vi "InitializeAllConfigs.vi"(10 "AllControlsRefs":T1, 11 "InstruConfig":T2={"Mode"="", "InstrumentMode"={"MainDAQ_Selector"=enum."None", "LaserCtrlMethod"=enum."SRS_DG535", "InstruMode"=enum."fsLDPI"}, "CommuniationSettings"={"SDG_II"="", "DG535"="", "BNC565"="", "EPM2000"="", "NI-DAQmx"="", "Micos"={"Simulation"=FALSE, "ComPort"="", "Serial Config"={"Baud Rate"=0, "Parity"=0, "Data Bits"=0, "Stop Bits"=0, "Flow Control"=0}, "#Axis"=0}, "ESP300"={"Simulation"=FALSE, "ComPort"="", "Serial Config"={"Baud Rate"=0, "Parity"=0, "Data Bits"=0, "Stop Bits"=0, "Flow Control"=0}, "#Axis"=0}}, "DG535"={"Trigger"={"Trigger Mode"=enum."Internal", "Internal/Burst Rate"=0.0, "External  Level"=0.0, "Impedance"=FALSE, "Slope"=FALSE}, "Delays"=[], "Output"=[]}, "Gage_Config"={"Acquisition"={"Sample Rate"=0.0, "Mode"=0, "Start (0)"=0.0, "Depth"=0.0, "Segment Size"=0.0, "Trigger Delay"=0.0, "Trigger Timeout"=0.0, "Trigger Holdoff"=0.0, "Clock mode"=enum."Internal", "Segment"=1}, "Channels"=[], "Trigger"={"Slope"=0, "Level"=0, "Source"=0, "External Range"=0, "External Coupling"=0, "External"=FALSE, "Disable"=FALSE, "External Impedance"=0}, "Mode(Gage)"=enum."Normal"}, "AnalogDisc_Config"={"Acqusition"={"Freq(Hz,SampleRate)"=0.0, "BufferSize"=0, "Mode"=enum."Single", "RecordLength(s)"=0.0}, "Channels"=[], "Trigger"={"TriggerSource"=enum."None", "Timeout(s)"=0.0, "Holdoff(s)"=0.0, "Position/Delay(s)"=0.0}, "AnalogTrigger"={"Channel"=0, "Polarity"=enum."Rising", "Type"=enum."Edge", "Level(V)"=0.0, "Filter"=enum."Decimate", "Hysterisis(V)"=0.0}}, "Micos"={"Velocity"=0.0, "Acceleration"=0.0}, "ESP300"={"Velocity"=[], "Acceleration"=[]}, "EPM2000"={"Factor(A)"=0.0, "Factor(B)"=0.0}, "ProcessMethod"={"TopLine"=0.0, "Threshold"=0.0, "Baseline"=0.0, "ZeroOffset"=0.0, "Processing Mode"=enum."None"}, "Timing(LDPI)"={"Delay(PI)"=0.0, "Delay(Rejection)"=0.0, "NoDelayOffset"=0.0, "RepRate(Hz)"=0.0}, "Cali."=[0.0707, 0.16163, 0.02539], "BNC_Config"={"System"={"Rep.Rate"=1000.0, "Sys Ext Mode"=enum."Triggered", "Mode"=enum."Single Shot"}, "Channels"=[]}} {"Cali." format="%#.6f"; "Timing(LDPI)"."Delay(PI)" format="%#_6p"; "Timing(LDPI)"."Delay(Rejection)" format="%#_6p"; "Timing(LDPI)"."NoDelayOffset" format="%#_6p"; "DG535"."Trigger"."External  Level" min=-2.56 max=2.56 format="%.2f"; "DG535"."Trigger"."Internal/Burst Rate" min=0.001 max=1000000.0 format="%.3f"; "DG535"."Delays"."Delay" format="%#_6p"; "DG535"."Output"."Offset" min=-3.0 max=4.0 format="%.2f"; "DG535"."Output"."Amplitude" min=-3.0 max=4.0 format="%.2f"; "ProcessMethod"."Threshold" format="%#_6p"; "Gage_Config"."Trigger"."External Impedance" items=["50 Ohm", "HiZ"]; "Gage_Config"."Trigger"."External Coupling" items=["DC", "AC"]; "Gage_Config"."Trigger"."External Range" min=2000 max=10000 step=8000; "Gage_Config"."Trigger"."Slope" items=["Rising", "Falling"]; "Gage_Config"."Trigger"."Level" min=-100 max=100; "Gage_Config"."Trigger"."Source" min=0 max=64 step=1; "Gage_Config"."Channels"."Impedance" min=50 max=1000000 step=999950; "Gage_Config"."Channels"."Coupling" items=["DC", "AC"]; "Gage_Config"."Acquisition"."Segment Size" min=256.0 step=128.0; "Gage_Config"."Acquisition"."Trigger Delay" min=0.0 step=128.0; "Gage_Config"."Acquisition"."Trigger Timeout" format="%.0p"; "Gage_Config"."Acquisition"."Trigger Holdoff" min=0.0 step=128.0; "Gage_Config"."Acquisition"."Depth" min=256.0 step=128.0; "Gage_Config"."Acquisition"."Mode" items=["Single", "Dual", "Quad", "Octal"]; "Gage_Config"."Acquisition"."Sample Rate" format="%.0p"; "AnalogDisc_Config"."AnalogTrigger"."Level(V)" format="%#_6p"; "AnalogDisc_Config"."AnalogTrigger"."Hysterisis(V)" format="%#_6p"; "AnalogDisc_Config"."Acqusition"."RecordLength(s)" format="%#_6p"; "AnalogDisc_Config"."Acqusition"."Freq(Hz,SampleRate)" format="%#_6p"; "AnalogDisc_Config"."Trigger"."Position/Delay(s)" format="%#_6p"; "AnalogDisc_Config"."Trigger"."Holdoff(s)" format="%#_6p"; "AnalogDisc_Config"."Trigger"."Timeout(s)" format="%#_6p"}) -> ()   [LabVIEW 2013]
uses:
  ControlDef/InstrumentConfiguration.ctl
  ControlDef/MainDAQ_Selector.ctl
  ControlDef/LaserCtrl_Method.ctl
  ControlDef/InstruMode_Typedef.ctl
  <instrlib>/DG535/Command/Set Trigger.ctl
  <instrlib>/DG535/Command/DG535_TriggerMode.ctl
  <instrlib>/DG535/Command/Set Delay.ctl
  <instrlib>/DG535/Command/DG535_Channel.ctl
  <instrlib>/DG535/Command/Set Output.ctl
  <instrlib>/DG535/Command/DG535_Output.ctl
  <instrlib>/GageLv_uic/VI/Gage_Configs.ctl
  <instrlib>/AnalogDiscSDKLv/VIs/DWF_AnalogIn_Configurations.ctl
  <instrlib>/AnalogDiscSDKLv/VIs/DWF_AcqMode.ctl
  <instrlib>/AnalogDiscSDKLv/VIs/DWF_Filter.ctl
  <instrlib>/AnalogDiscSDKLv/VIs/DWF_TrigSrc.ctl
  <instrlib>/AnalogDiscSDKLv/VIs/DWF_TrigCond.ctl
  <instrlib>/AnalogDiscSDKLv/VIs/DWF_TrigType.ctl
  ControlDef/ProcessingMode.ctl
  <instrlib>/BNC/Public/BNC_Configs.ctl
  ControlDef/InstrumentSpecificControls/UIC-AToF/InitializationParams_BNC565_2Ch_AToF.ctl
  Hardware/BNC(QuantumComposers)/Command/Set C-Input.ctl
  Hardware/BNC(QuantumComposers)/Command/Set C-Mode.ctl
  Hardware/BNC(QuantumComposers)/Command/Set C-Output.ctl
  Hardware/BNC(QuantumComposers)/Command/Set C-Enable.ctl
  ControlDef/AllControlsRefs.ctl
  <instrlib>/DG535/SRS_DG535_Lib.lvlib
  <instrlib>/GageLv_uic/Gage.lvlib
  <instrlib>/AnalogDiscSDKLv/AnalogDiscSDKLv.lvlib
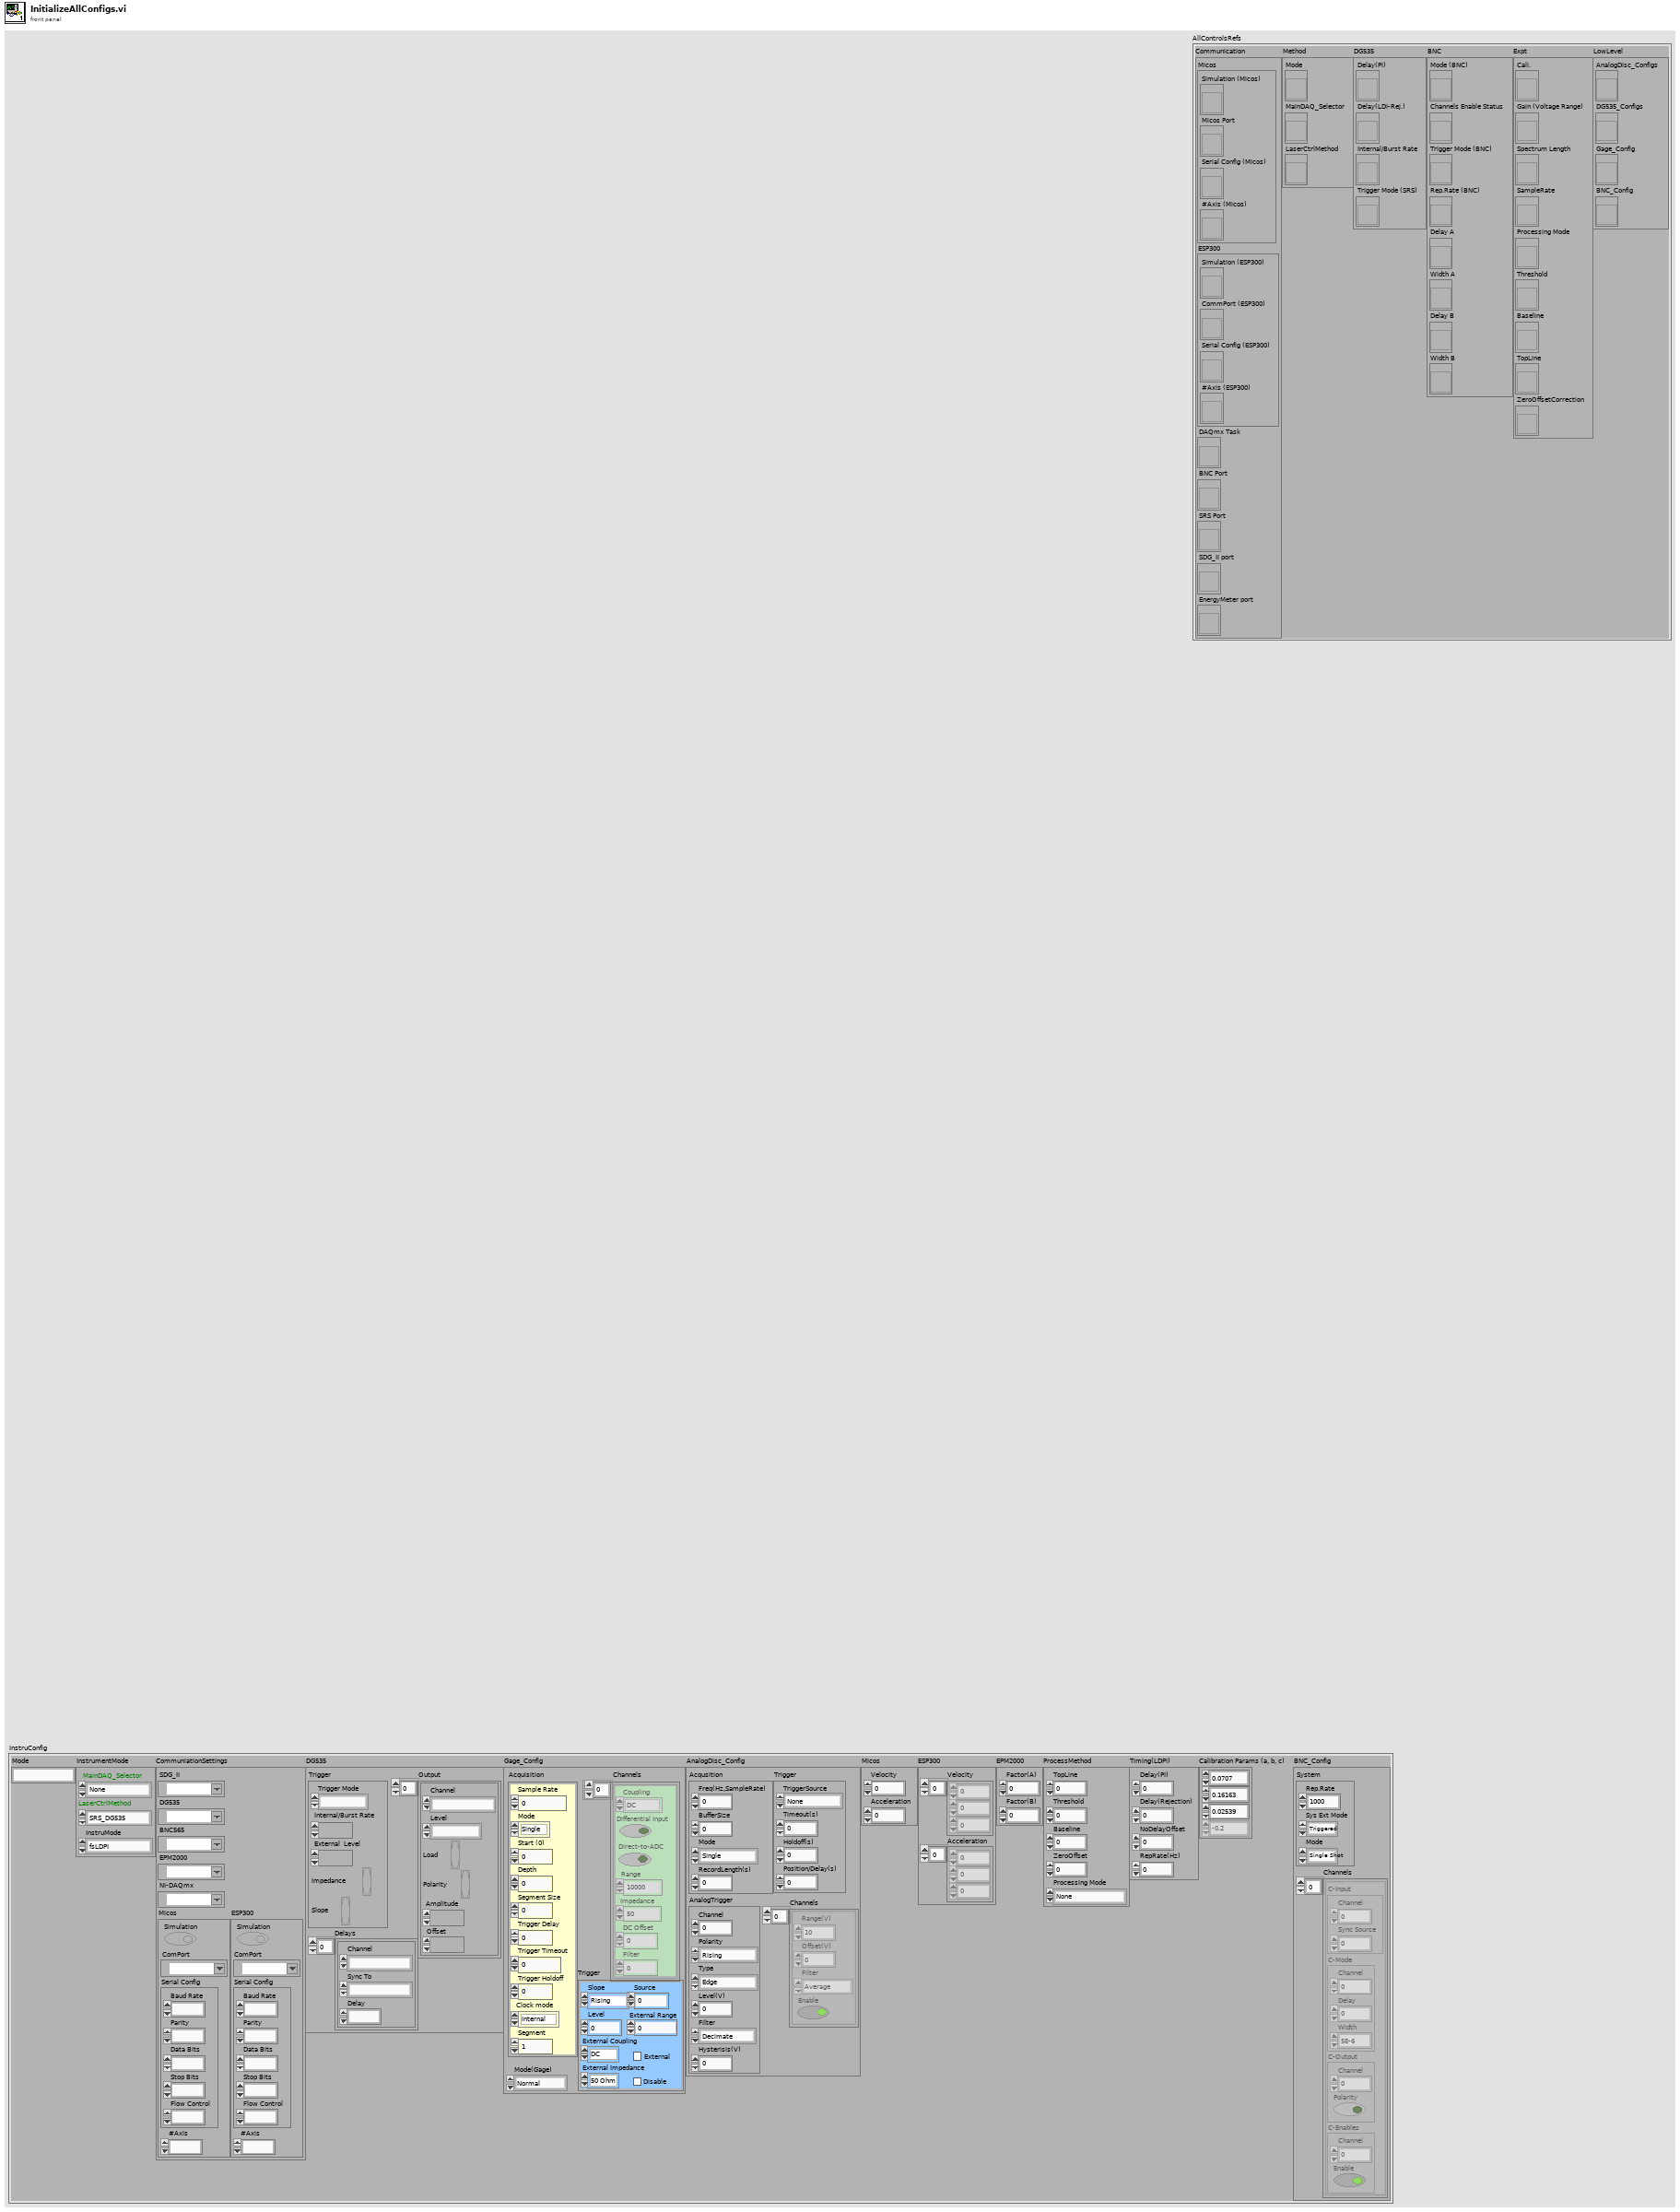
[diagram p1: front panel]
types:
  T1 = typedef "AllControlsRefs.ctl" = cluster{"Communication":cluster{"Micos":cluster{"Simulation (Micos)":refnum<vi>, "Micos Port":refnum<vi>, "Serial Config (Micos)":refnum<vi>, "#Axis (Micos)":refnum<vi>}, "ESP300":cluster{"Simulation (ESP300)":refnum<vi>, "CommPort (ESP300)":refnum<vi>, "Serial Config (ESP300)":refnum<vi>, "#Axis (ESP300)":refnum<vi>}, "DAQmx Task":refnum<vi>, "BNC Port":refnum<vi>, "SRS Port":refnum<vi>, "SDG_II port":refnum<vi>, "EnergyMeter port":refnum<vi>}, "Method":cluster{"Mode":refnum<vi>, "MainDAQ_Selector":refnum<vi>, "LaserCtrlMethod":refnum<vi>}, "DG535":cluster{"Delay(PI)":refnum<vi>, "Delay(LDI-Rej.)":refnum<vi>, "Internal/Burst Rate":refnum<vi>, "Trigger Mode (SRS)":refnum<vi>}, "BNC":cluster{"Mode (BNC)":refnum<vi>, "Channels Enable Status":refnum<vi>, "Trigger Mode (BNC)":refnum<vi>, "Rep.Rate (BNC)":refnum<vi>, "Delay A":refnum<vi>, "Width A":refnum<vi>, "Delay B":refnum<vi>, "Width B":refnum<vi>}, "Expt":cluster{"Cali.":refnum<vi>, "Gain (Voltage Range)":refnum<vi>, "Spectrum Length":refnum<vi>, "SampleRate":refnum<vi>, "Processing Mode":refnum<vi>, "Threshold":refnum<vi>, "Baseline":refnum<vi>, "TopLine":refnum<vi>, "ZeroOffsetCorrection":refnum<vi>}, "LowLevel":cluster{"AnalogDisc_Configs":refnum<vi>, "DG535_Configs":refnum<vi>, "Gage_Config":refnum<vi>, "BNC_Config":refnum<vi>}}
  T2 = typedef "InstrumentConfiguration.ctl" = cluster{"Mode":string, "InstrumentMode":cluster{"MainDAQ_Selector":T3, "LaserCtrlMethod":T4, "InstruMode":T5}, "CommuniationSettings":cluster{"SDG_II":refnum<visa-resource-name>, "DG535":refnum<visa-resource-name>, "BNC565":refnum<visa-resource-name>, "EPM2000":refnum<visa-resource-name>, "NI-DAQmx":refnum<visa-resource-name>, "Micos":cluster{"Simulation":bool, "ComPort":refnum<visa-resource-name>, "Serial Config":cluster{"Baud Rate":u32, "Parity":u16, "Data Bits":u16, "Stop Bits":u16, "Flow Control":u16}, "#Axis":i32}, "ESP300":cluster{"Simulation":bool, "ComPort":refnum<visa-resource-name>, "Serial Config":cluster{"Baud Rate":u32, "Parity":u16, "Data Bits":u16, "Stop Bits":u16, "Flow Control":u16}, "#Axis":i32}}, "DG535":cluster{"Trigger":T6, "Delays":T8[], "Output":T10[]}, "Gage_Config":T12, "AnalogDisc_Config":T13, "Micos":cluster{"Velocity":dbl, "Acceleration":dbl}, "ESP300":cluster{"Velocity":dbl[], "Acceleration":dbl[]}, "EPM2000":cluster{"Factor(A)":dbl, "Factor(B)":dbl}, "ProcessMethod":cluster{"TopLine":dbl, "Threshold":dbl, "Baseline":dbl, "ZeroOffset":dbl, "Processing Mode":T19}, "Timing(LDPI)":cluster{"Delay(PI)":dbl, "Delay(Rejection)":dbl, "NoDelayOffset":dbl, "RepRate(Hz)":dbl}, "Cali.":dbl[], "BNC_Config":T20}
  T3 = typedef "MainDAQ_Selector.ctl" = enum16{"None", "Gage", "Gage_Double", "IonWerks_TDCx4", "Tektronics", "KnifeEdge_Emu", "AnalogDisc"}
  T4 = typedef "LaserCtrl_Method.ctl" = enum16{"SRS_DG535", "BNC", "SDG_II"}
  T5 = typedef "InstruMode_Typedef.ctl" = enum16{"fsLDPI", "nsLDPI", "nsLD-fsPI", "GenericTOF", "BeamProfiling"}
  T6 = typedef "SRS_DG535_Lib.lvlib/Set Trigger.ctl" = cluster{"Trigger Mode":T7, "Internal/Burst Rate":dbl, "External  Level":sgl, "Impedance":bool, "Slope":bool}
  T7 = typedef "SRS_DG535_Lib.lvlib/DG535_TriggerMode.ctl" = enum16{"Internal", "External", "SingleShot", "Burst", "Line"}
  T8 = typedef "SRS_DG535_Lib.lvlib/Set Delay.ctl" = cluster{"Channel":T9, "Sync To":T9, "Delay":dbl}
  T9 = typedef "SRS_DG535_Lib.lvlib/DG535_Channel.ctl" = enum16{"Trigger Input", "T0 Output", "A Output", "B Output", "AB Output", "C Output", "D Output", "CD Output", "NULL"}
  T10 = typedef "SRS_DG535_Lib.lvlib/Set Output.ctl" = cluster{"Channel":T9, "Level":T11, "Load":bool, "Polarity":bool, "Amplitude":dbl, "Offset":dbl}
  T11 = typedef "SRS_DG535_Lib.lvlib/DG535_Output.ctl" = enum16{"TTL", "NIM", "ECL", "Variable"}
  T12 = typedef "Gage.lvlib/Gage_Configs.ctl" = cluster{"Acquisition":cluster{"Sample Rate":dbl, "Mode":u16, "Start (0)":dbl, "Depth":dbl, "Segment Size":dbl, "Trigger Delay":dbl, "Trigger Timeout":dbl, "Trigger Holdoff":dbl, "Clock mode":enum16{"Internal", "External", "Reference"}, "Segment":u32}, "Channels":cluster{"Coupling":u16, "Differential Input":bool, "Direct-to-ADC":bool, "Range":u32, "Impedance":u32, "DC Offset":i32, "Filter":i32}[], "Trigger":cluster{"Slope":u16, "Level":i32, "Source":i32, "External Range":u32, "External Coupling":u16, "External":bool, "Disable":bool, "External Impedance":u16}, "Mode(Gage)":enum16{"Normal", "Continuous", "MultiRecord", "HwAverage"}}
  T13 = typedef "AnalogDiscSDKLv.lvlib/DWF_AnalogIn_Configurations.ctl" = cluster{"Acqusition":cluster{"Freq(Hz,SampleRate)":dbl, "BufferSize":i32, "Mode":T14, "RecordLength(s)":dbl}, "Channels":cluster{"Range(V)":dbl, "Offset(V)":dbl, "Filter":T15, "Enable":bool}[], "Trigger":cluster{"TriggerSource":T16, "Timeout(s)":dbl, "Holdoff(s)":dbl, "Position/Delay(s)":dbl}, "AnalogTrigger":cluster{"Channel":i32, "Polarity":T17, "Type":T18, "Level(V)":dbl, "Filter":T15, "Hysterisis(V)":dbl}}
  T14 = typedef "AnalogDiscSDKLv.lvlib/DWF_AcqMode.ctl" = enum16{"Single", "ScanShift", "ScanScreen", "Record"}
  T15 = typedef "AnalogDiscSDKLv.lvlib/DWF_Filter.ctl" = enum16{"Decimate", "Average", "MinMax"}
  T16 = typedef "AnalogDiscSDKLv.lvlib/DWF_TrigSrc.ctl" = enum16{"None", "PC", "DetectorAnalogIn", "DetectorDigitalIn", "AnalogIn", "DigitalIn", "DigitalOut", "AnalogOut1", "AnalogOut2", "AnalogOut3", "AnalogOut4", "External1", "External2", "External3", "External4"}
  T17 = typedef "AnalogDiscSDKLv.lvlib/DWF_TrigCond.ctl" = enum16{"Rising", "Falling"}
  T18 = typedef "AnalogDiscSDKLv.lvlib/DWF_TrigType.ctl" = enum16{"Edge", "Pulse", "Transition"}
  T19 = typedef "ProcessingMode.ctl" = enum16{"None", "Drop by Threshold", "TDC Simulate", "SetFilter"}
  T20 = typedef "BNC_Configs.ctl" = cluster{"System":cluster{"Rep.Rate":dbl, "Sys Ext Mode":enum16{"Disabled", "Triggered", "Gated", "Triggered & Gated"}, "Mode":enum16{"Normal", "Single Shot", "Duty Cycle", "Burst"}}, "Channels":T21[]}
  T21 = typedef "InitializationParams_BNC565_2Ch_AToF.ctl" = cluster{"C-Input":T22, "C-Mode":T23, "C-Output":T24, "C-Enables":T25}
  T22 = typedef "Set C-Input.ctl" = cluster{"Channel":i32, "Sync Source":i32}
  T23 = typedef "Set C-Mode.ctl" = cluster{"Channel":i32, "Delay":dbl, "Width":dbl}
  T24 = typedef "Set C-Output.ctl" = cluster{"Channel":i32, "Polarity":bool}
  T25 = typedef "Set C-Enable.ctl" = cluster{"Channel":i32, "Enable":bool}
  T26 = enum16{"Disabled", "Triggered", "Gated", "Triggered & Gated"}
  T27 = enum16{"Normal", "Single Shot", "Duty Cycle", "Burst"}
  T28 = cluster{"Trigger":T6, "Delays":T8[], "Output":T10[]}
  T29 = cluster{"Baud Rate":u32, "Parity":u16, "Data Bits":u16, "Stop Bits":u16, "Flow Control":u16}
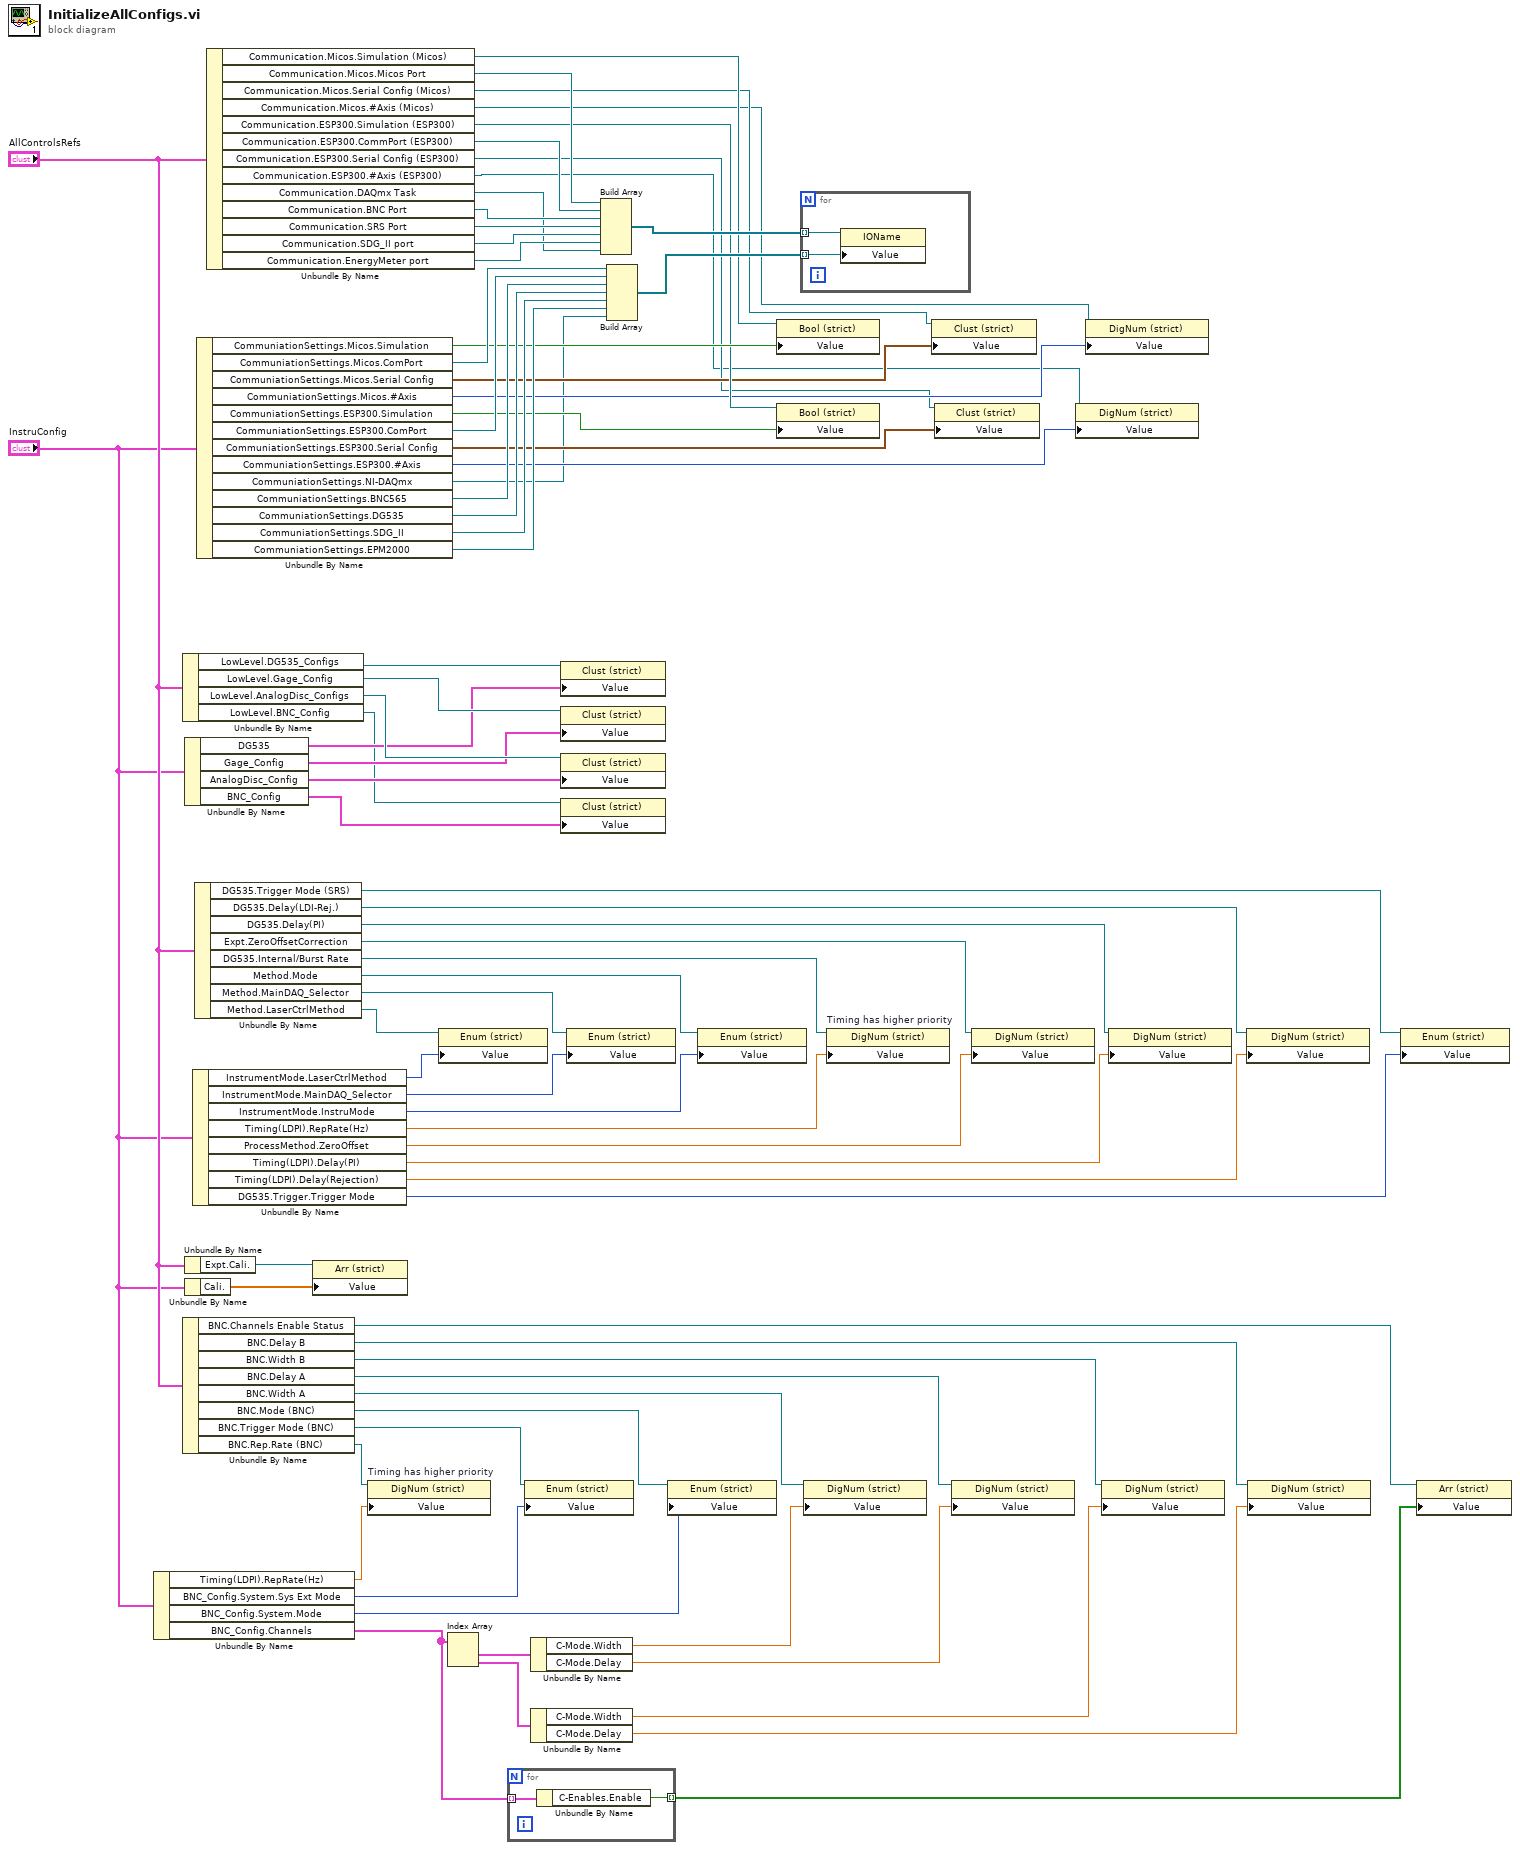
[diagram p0: block diagram]
diagram:
  n1 = Unbundle By Name("InstruConfig") -> ("Timing(LDPI).RepRate(Hz)"=w19:dbl, "BNC_Config.System.Sys Ext Mode"=w16:T26, "BNC_Config.System.Mode"=w14:T27, "BNC_Config.Channels"=w3:T21[])
  n2 = Unbundle By Name("AllControlsRefs") -> ("LowLevel.DG535_Configs"=w61:refnum<vi>, "LowLevel.Gage_Config"=w60:refnum<vi>, "LowLevel.AnalogDisc_Configs"=w59:refnum<vi>, "LowLevel.BNC_Config"=w23:refnum<vi>)
  n3 = Unbundle By Name("AllControlsRefs") -> ("BNC.Channels Enable Status"=w2:refnum<vi>, "BNC.Delay B"=w9:refnum<vi>, "BNC.Width B"=w10:refnum<vi>, "BNC.Delay A"=w11:refnum<vi>, "BNC.Width A"=w12:refnum<vi>, "BNC.Mode (BNC)"=w15:refnum<vi>, "BNC.Trigger Mode (BNC)"=w17:refnum<vi>, "BNC.Rep.Rate (BNC)"=w18:refnum<vi>)
  n4 = Unbundle By Name("InstruConfig") -> ("DG535"=w58:T28, "Gage_Config"=w57:T12, "AnalogDisc_Config"=w56:T13, "BNC_Config"=w22:T20)
  n5 = Unbundle By Name("AllControlsRefs") -> ("Expt.Cali."=w25:refnum<vi>)
  n6 = Unbundle By Name("InstruConfig") -> ("Cali."=w24:dbl[])
  n7 = Unbundle By Name("InstruConfig") -> ("InstrumentMode.LaserCtrlMethod"=w38:T4, "InstrumentMode.MainDAQ_Selector"=w37:T3, "InstrumentMode.InstruMode"=w36:T5, "Timing(LDPI).RepRate(Hz)"=w34:dbl, "ProcessMethod.ZeroOffset"=w32:dbl, "Timing(LDPI).Delay(PI)"=w28:dbl, "Timing(LDPI).Delay(Rejection)"=w27:dbl, "DG535.Trigger.Trigger Mode"=w26:T7)
  n8 = Unbundle By Name("AllControlsRefs") -> ("DG535.Trigger Mode (SRS)"=w29:refnum<vi>, "DG535.Delay(LDI-Rej.)"=w30:refnum<vi>, "DG535.Delay(PI)"=w31:refnum<vi>, "Expt.ZeroOffsetCorrection"=w33:refnum<vi>, "DG535.Internal/Burst Rate"=w35:refnum<vi>, "Method.Mode"=w41:refnum<vi>, "Method.MainDAQ_Selector"=w40:refnum<vi>, "Method.LaserCtrlMethod"=w39:refnum<vi>)
  n9 = Unbundle By Name("InstruConfig") -> ("CommuniationSettings.Micos.Simulation"=w54:bool, "CommuniationSettings.Micos.ComPort"=w68:refnum<visa-resource-name>, "CommuniationSettings.Micos.Serial Config"=w49:T29, "CommuniationSettings.Micos.#Axis"=w48:i32, "CommuniationSettings.ESP300.Simulation"=w53:bool, "CommuniationSettings.ESP300.ComPort"=w67:refnum<visa-resource-name>, "CommuniationSettings.ESP300.Serial Config"=w45:T29, "CommuniationSettings.ESP300.#Axis"=w44:i32, "CommuniationSettings.NI-DAQmx"=w42:refnum<visa-resource-name>, "CommuniationSettings.BNC565"=w66:refnum<visa-resource-name>, "CommuniationSettings.DG535"=w65:refnum<visa-resource-name>, "CommuniationSettings.SDG_II"=w64:refnum<visa-resource-name>, "CommuniationSettings.EPM2000"=w63:refnum<visa-resource-name>)
  n10 = Unbundle By Name("AllControlsRefs") -> ("Communication.Micos.Simulation (Micos)"=w55:refnum<vi>, "Communication.Micos.Micos Port"=w75:refnum<vi>, "Communication.Micos.Serial Config (Micos)"=w51:refnum<vi>, "Communication.Micos.#Axis (Micos)"=w50:refnum<vi>, "Communication.ESP300.Simulation (ESP300)"=w52:refnum<vi>, "Communication.ESP300.CommPort (ESP300)"=w74:refnum<vi>, "Communication.ESP300.Serial Config (ESP300)"=w47:refnum<vi>, "Communication.ESP300.#Axis (ESP300)"=w46:refnum<vi>, "Communication.DAQmx Task"=w43:refnum<vi>, "Communication.BNC Port"=w73:refnum<vi>, "Communication.SRS Port"=w72:refnum<vi>, "Communication.SDG_II port"=w71:refnum<vi>, "Communication.EnergyMeter port"=w70:refnum<vi>)
  n11 = property class="Arr (strict)"(reference=w25, "Value"=w24) -> ()  [unwired: 1 in, 2 out]
  n12 = property on="Timing has higher priority" class="DigNum (strict)"(reference=w18, "Value"=w19) -> ()  [unwired: 1 in, 2 out]
  n13 = property class="Enum (strict)"(reference=w39, "Value"=w38) -> ()  [unwired: 1 in, 2 out]
  n14 = Index Array(array=w3) -> (element #1=w13:T21, element #2=w6:T21)  [unwired: 2 in]
  n15 = for {
    tunnel: w3 -> [w77] mode=indexing
    tunnel: [w76] -> w1 mode=indexing
    n16 = Unbundle By Name(w77) -> ("C-Enables.Enable"=w76:bool)
  }
  n17 = property class="Enum (strict)"(reference=w17, "Value"=w16) -> ()  [unwired: 1 in, 2 out]
  n18 = Unbundle By Name(w13) -> ("C-Mode.Width"=w8:dbl, "C-Mode.Delay"=w7:dbl)
  n19 = Unbundle By Name(w6) -> ("C-Mode.Width"=w5:dbl, "C-Mode.Delay"=w4:dbl)
  n20 = property class="Clust (strict)"(reference=w61, "Value"=w58) -> ()  [unwired: 1 in, 2 out]
  n21 = property class="Clust (strict)"(reference=w60, "Value"=w57) -> ()  [unwired: 1 in, 2 out]
  n22 = property class="Clust (strict)"(reference=w59, "Value"=w56) -> ()  [unwired: 1 in, 2 out]
  n23 = property class="Clust (strict)"(reference=w23, "Value"=w22) -> ()  [unwired: 1 in, 2 out]
  n24 = property class="Enum (strict)"(reference=w40, "Value"=w37) -> ()  [unwired: 1 in, 2 out]
  n25 = Build Array(w75, w74, w73, w72, w71, w70, w43) -> (w69:refnum<vi>[])
  n26 = Build Array(w68, w67, w66, w65, w64, w63, w42) -> (w62:refnum<visa-resource-name>[])
  n27 = property class="Enum (strict)"(reference=w15, "Value"=w14) -> ()  [unwired: 1 in, 2 out]
  n28 = property class="Enum (strict)"(reference=w41, "Value"=w36) -> ()  [unwired: 1 in, 2 out]
  n29 = property class="Bool (strict)"(reference=w55, "Value"=w54) -> ()  [unwired: 1 in, 2 out]
  n30 = property class="Bool (strict)"(reference=w52, "Value"=w53) -> ()  [unwired: 1 in, 2 out]
  n31 = for {
    tunnel: w69 -> [w79] mode=indexing
    tunnel: w62 -> [w78] mode=indexing
    n32 = property class="IOName"(reference=w79, "Value"=w78) -> ()  [unwired: 1 in, 2 out]
  }
  n33 = property class="DigNum (strict)"(reference=w12, "Value"=w8) -> ()  [unwired: 1 in, 2 out]
  n34 = property on="Timing has higher priority" class="DigNum (strict)"(reference=w35, "Value"=w34) -> ()  [unwired: 1 in, 2 out]
  n35 = property class="Clust (strict)"(reference=w51, "Value"=w49) -> ()  [unwired: 1 in, 2 out]
  n36 = property class="Clust (strict)"(reference=w47, "Value"=w45) -> ()  [unwired: 1 in, 2 out]
  n37 = property class="DigNum (strict)"(reference=w11, "Value"=w7) -> ()  [unwired: 1 in, 2 out]
  n38 = property class="DigNum (strict)"(reference=w33, "Value"=w32) -> ()  [unwired: 1 in, 2 out]
  n39 = property class="DigNum (strict)"(reference=w46, "Value"=w44) -> ()  [unwired: 1 in, 2 out]
  n40 = property class="DigNum (strict)"(reference=w50, "Value"=w48) -> ()  [unwired: 1 in, 2 out]
  n41 = property class="DigNum (strict)"(reference=w10, "Value"=w5) -> ()  [unwired: 1 in, 2 out]
  n42 = property class="DigNum (strict)"(reference=w31, "Value"=w28) -> ()  [unwired: 1 in, 2 out]
  n43 = property class="DigNum (strict)"(reference=w30, "Value"=w27) -> ()  [unwired: 1 in, 2 out]
  n44 = property class="DigNum (strict)"(reference=w9, "Value"=w4) -> ()  [unwired: 1 in, 2 out]
  n45 = property class="Enum (strict)"(reference=w29, "Value"=w26) -> ()  [unwired: 1 in, 2 out]
  n46 = property class="Arr (strict)"(reference=w2, "Value"=w1) -> ()  [unwired: 1 in, 2 out]
